vi "ModeloPrimerOrden.vi"() -> ()   [LabVIEW 2019]
uses:
  <vilib>/addons/Control Design/_Model Construction/Special Model Creation.llb/Special Model Creation SubVI/CD Create 1st Order Model.vi
  <vilib>/addons/Control Design/_Utility/Model Viewer.llb/Model Viewer SubVI/cd_Draw Transfer Function Equation (TF).vi
  <vilib>/addons/control/pid/pid.llb/PID (DBL).vi
  <vilib>/addons/control/pid/NI_PID_pid.lvlib
  <vilib>/addons/Control Design/_Model Construction/NI_CD_Special Model Creation.lvlib
  <vilib>/addons/Control Design/_Utility/NI_CD_Model Viewer.lvlib
panel:
  out "Equation":picture
  in  "Tau":dbl
  in  "K":dbl=1.0
  out "Waveform Chart":T1(graph)
  in  "input cluster":T1
  in  "setpoint":dbl format="%#_13g"
  in  "PID gains":T2={"proportional gain (Kc)"=1.0, "integral time (Ti, min)"=0.01, "derivative time (Td, min)"=0.0} {"derivative time (Td, min)" format="%.3f"; "integral time (Ti, min)" format="%.3f"; "proportional gain (Kc)" format="%.3f"}
  in  "paso (s)":dbl
  in  "stop":bool
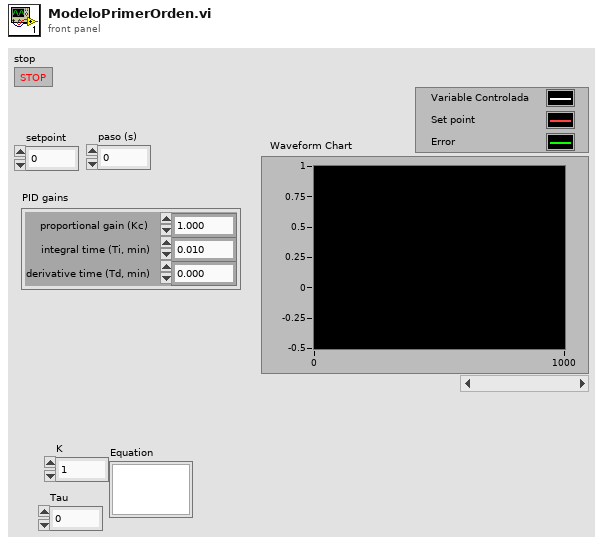
[diagram p1: front panel]
types:
  T1 = cluster{"Variable controlada":dbl, "Set Point":dbl, "Error":dbl}
  T2 = cluster{"proportional gain (Kc)":dbl, "integral time (Ti, min)":dbl, "derivative time (Td, min)":dbl}
  T3 = typedef "NI_LinSys_Model Typedefs.lvlib/CD Transfer Function Model (MIMO).ctl" = cluster{"properties":T4, "transfer function(s)":T5[][]}
  T4 = typedef "NI_LinSys_Model Typedefs.lvlib/CD General Elements.ctl" = cluster{"Model name":string, "Input names":string[], "Output names":string[], "Input Delays":dbl[], "Output Delays":dbl[], "Sampling Time":dbl, "Notes":string}
  T5 = typedef "NI_LinSys_Model Typedefs.lvlib/CD Transfer Function Model (SISO).ctl" = cluster{"Numerator":dbl[], "Denominator":dbl[], "delay":dbl}
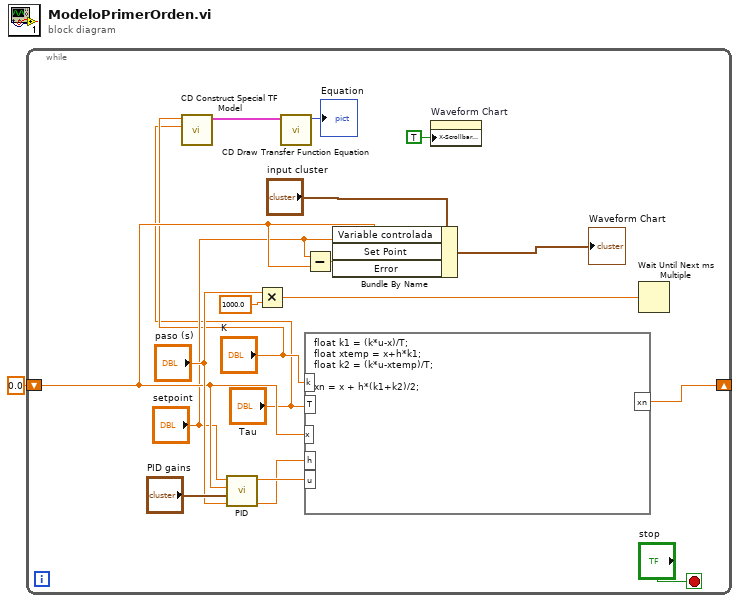
[diagram p0: block diagram]
diagram:
  n1 = while {
    shift-right: [w16] -> _
    shift-left: 0.0 ("xn") -> [w11]
    stop <- "stop" stop-if-true
    n2 = call-poly <vilib>:"CD Construct Special TF Model.vi"("Time Constant (s)"="Tau", "Static Gain"="K") -> ("Transfer Function Model"=w3:T3)  [unwired: 8 in, 1 out]
    n3 = call-poly <vilib>:"PID.vi"("dt (s)"="paso (s)", "PID gains"="PID gains", "process variable"=w11, "setpoint"="setpoint") -> ("dt out (s)"=w12:dbl, "output"=w17:dbl)  [unwired: 6 in]
    n4 = Multiply(x="paso (s)", y=1000.0) -> (x*y=w13:dbl)
    n5 = call-poly <vilib>:"CD Draw Transfer Function Equation.vi"("Transfer Function Model"=w3) -> ("Equation"=→"Equation":picture)  [unwired: 8 in, 2 out]
    n6 = Subtract(x="setpoint", y=w11) -> (x-y=w9:dbl)
    n7 = formula code="float k1 = (k*u-x)/T;\nfloat xtemp = x+h*k1;\nfloat k2 = (k*u-xtemp)/T;\n\nxn = x + h*(k1+k2)/2;"("k"="K", "T"="Tau", "x"=w11, "h"=w12, "u"=w17) -> ("xn"=w16:dbl)
    n8 = Bundle By Name(cluster="input cluster", "Variable controlada"=w11, "Set Point"="setpoint", "Error"=w9) -> (→"Waveform Chart":T1)
    n9 = property on="Waveform Chart" class="WFChart (strict)"("X-Scrollbar Visible"=TRUE ("X Scrollbar Visible")) -> ()  [unwired: 2 in, 2 out]
    n10 = Wait Until Next ms Multiple(millisecond multiple=w13) -> ()  [unwired: 1 out]
  }
